vi "SUB_RTXDll_Read.vi"(3 "CMD":string) -> (1 "OUTPUT":string)   [LabVIEW 2011]
uses:
  R2012dll.dll
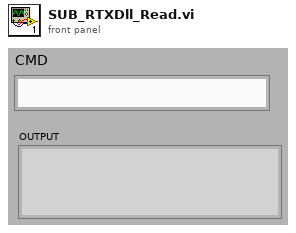
[diagram p1: front panel]
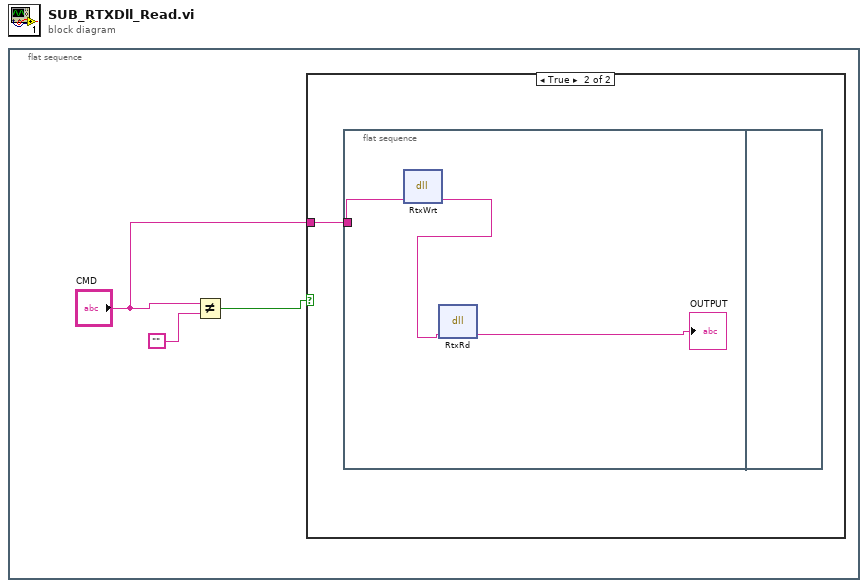
[diagram p0: block diagram]
diagram:
  n1 = flat-sequence {
    frame #0 {
      n2 = Not Equal?(x="CMD", y="") -> (x != y?=w2:bool)
      n3 = case shown="True" w2 {
        tunnel: "CMD" -> [_ w4]
        frame False {
        }
        frame True {
          n4 = flat-sequence {
            tunnel: w4 -> [w7]
            frame #0 {
              n5 = dll-call lib="E:/Konftel_Project/R2012dll.dll" fn="RtxWrt"("RtxWrt"=w7) -> ("RtxWrt"=w6:string)  [unwired: 4 in, 2 out]
              n6 = dll-call lib="E:/Konftel_Project/R2012dll.dll" fn="RtxRd"("RtxRd"=w6) -> ("RtxRd"=→"OUTPUT":string)  [unwired: 4 in, 2 out]
            }
            frame #1 {
            }
          }
        }
      }
    }
  }
